vi "Go Straight.vi"(0 "VISA resource name in":refnum<visa-resource-name>, 1 "Sequence Active":bool, 2 "Current sequence":string[](array[string]), 3 "Speed":dbl(knob) scale=0.0..20.0, 4 "Steps(mm)":dbl[](array[numeric]), 5 "error in":errorcluster) -> (6 "VISA resource name out":refnum<visa-resource-name>, 7 "Koordinaten IF6":T1 {"Schritte B" format="%#.4g"; "Schritte A" format="%#.4g"; "Schritte C" format="%#.4g"; "Schritte U" format="%#.4g"; "Schritte Z" format="%#.4g"; "Schritte Y" format="%#.4g"; "Schritte X" format="%#.4g"}, 8 "error out":errorcluster)   [LabVIEW 2013]
panel:
  in  "Schritte oder mm (mm)":u16(ring) items=["Schritte", "mm"]
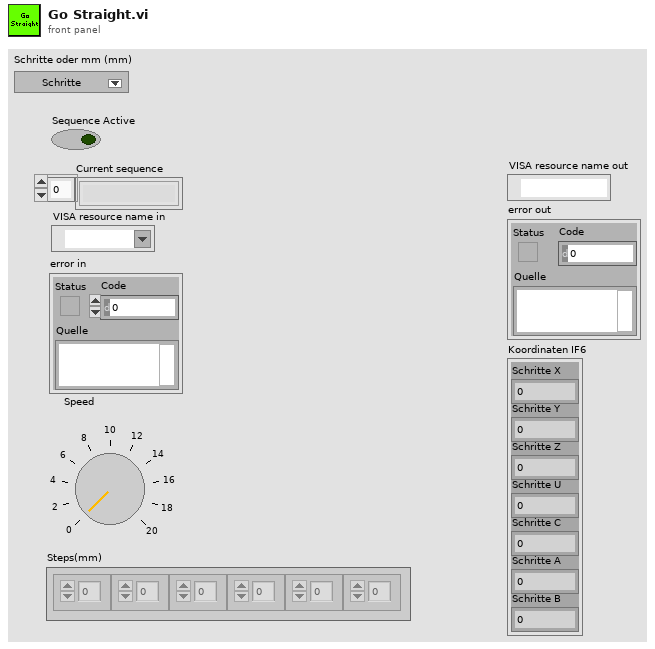
[diagram p1: front panel]
types:
  T1 = cluster{"Schritte X":sgl, "Schritte Y":sgl, "Schritte Z":sgl, "Schritte U":sgl, "Schritte C":sgl, "Schritte A":sgl, "Schritte B":sgl}
  T2 = cluster{"[0]":dbl, "[1]":dbl, "[2]":dbl, "[3]":dbl, "[4]":dbl, "[5]":dbl, "[6]":dbl, "[7]":dbl, "[8]":dbl}
  T3 = enum16{"vom Endschalter weg", "zum Endschalter hin"}
  T4 = cluster{enum16{"vom Endschalter weg", "zum Endschalter hin"}, enum16{"vom Endschalter weg", "zum Endschalter hin"}, enum16{"vom Endschalter weg", "zum Endschalter hin"}}
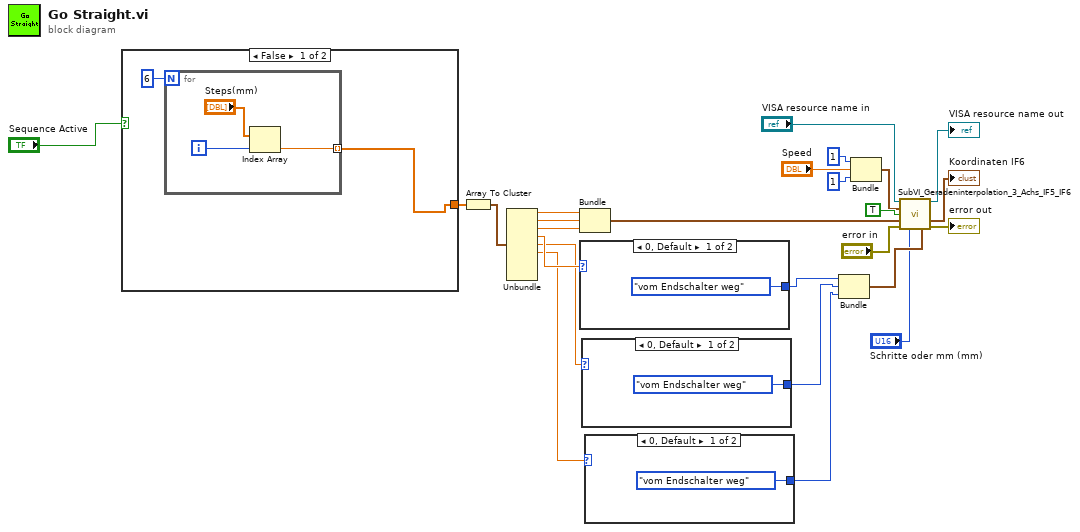
[diagram p0: block diagram]
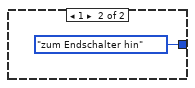
[diagram p2: hidden frame]
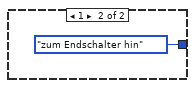
[diagram p3: hidden frame]
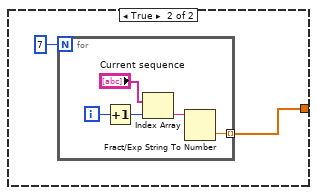
[diagram p4: hidden frame]
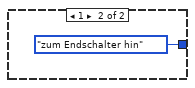
[diagram p5: hidden frame]
diagram:
  n1 = case shown="False" "Sequence Active" {
    tunnel: [w26 w31] -> w9
    frame False {
      n2 = for {
        N: 6 -> [_]
        tunnel: [w29] -> w26 mode=indexing
        i -> [w28]
        n3 = Index Array(array="Steps(mm)", index=w28) -> (element=w29:dbl)
      }
    }
    frame True {
      n4 = for {
        N: 7 -> [_]
        tunnel: [w33] -> w31 mode=indexing
        i -> [w34]
        n5 = Increment(x=w34) -> (x+1=w37:i32)
        n6 = Index Array(array="Current sequence", index=w37) -> (element=w36:string)
        n7 = Fract/Exp String To Number(string=w36) -> (number=w33:dbl)  [unwired: 3 in, 1 out]
      }
    }
  }
  n8 = Array To Cluster(array=w9) -> (cluster=w8:T2)
  n9 = Unbundle(w8) -> ("[0]"=w25:dbl, "[1]"=w24:dbl, "[2]"=w23:dbl, "[3]"=w7:dbl, "[4]"=w6:dbl, "[5]"=w5:dbl)  [unwired: 3 out]
  n10 = Bundle("[0]"=w25, "[1]"=w24, "[2]"=w23) -> (w15:cluster{"[0]":dbl, "[1]":dbl, "[2]":dbl})  [unwired: 1 in]
  n11 = case shown="0, Default" w7 {
    tunnel: [T3."vom Endschalter weg" T3."zum Endschalter hin"] -> w4
    frame 0, Default {
    }
    frame 1 {
    }
  }
  n12 = case shown="0, Default" w6 {
    tunnel: [T3."vom Endschalter weg" T3."zum Endschalter hin"] -> w3
    frame 0, Default {
    }
    frame 1 {
    }
  }
  n13 = case shown="0, Default" w5 {
    tunnel: [T3."vom Endschalter weg" T3."zum Endschalter hin"] -> w2
    frame 0, Default {
    }
    frame 1 {
    }
  }
  n14 = Bundle(w4, w3, w2) -> (w22:T4)  [unwired: 1 in]
  n15 = Bundle(1, "Speed"="Speed", 1) -> (w14:cluster{i32, "Speed":dbl, i32})  [unwired: 1 in]
  n16 = call <userlib>:"SubVI_Geradeninterpolation_3_Achs_IF5_IF6.vi"("VISA resource name in"="VISA resource name in", "Geschwindigkeiten"=w14, "IF5=F/IF6=T\n(IF6=T) in"=TRUE ("IF5=F/IF6=T\n(IF6=T) in"), "Abstände"=w15, "error in"="error in", "Schritte oder mm (mm)"="Schritte oder mm (mm)", "Richtungen"=w22) -> ("VISA resource name out"=→"VISA resource name out":refnum<visa-resource-name>, "Koordinaten IF6"=→"Koordinaten IF6":T1, "error out"=→"error out":errorcluster)  [unwired: 3 in, 3 out]
